vi "Logger Write To File.vi"(0 "Log File Input":T1, 11 "error in (no error)":errorcluster) -> (15 "error out":errorcluster)   [LabVIEW 2018]
uses:
  Logger Global.vi
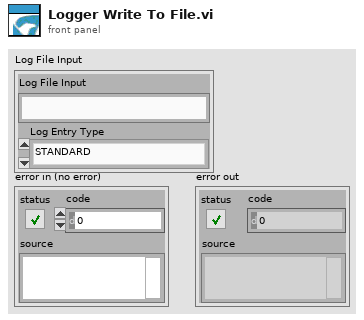
[diagram p1: front panel]
types:
  T1 = cluster{"Log File Input":string, "Log Entry Type":enum16{"STANDARD", "WARNING", "CRITICAL"}}
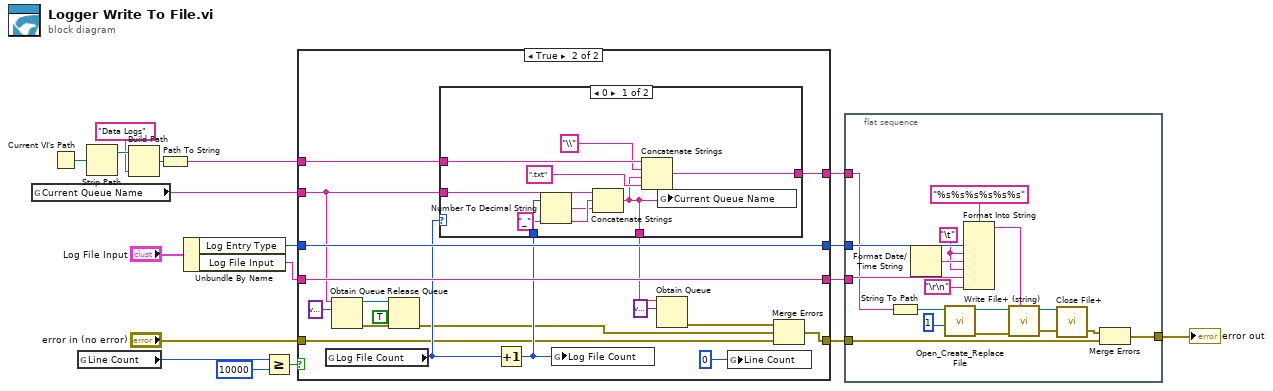
[diagram p0: block diagram]
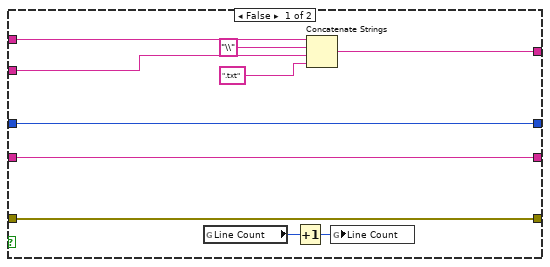
[diagram p2: hidden frame]
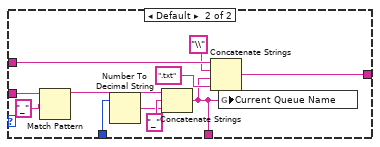
[diagram p3: hidden frame]
diagram:
  n1 = global read "Logger Global.vi" "Current Queue Name"() -> (w2:string)
  n2 = Current VI's Path() -> (path=w7:path)
  n3 = global read "Logger Global.vi" "Line Count"() -> (w10:u16)
  n4 = Strip Path(path=w7) -> (stripped path=w6:path)  [unwired: 1 out]
  n5 = Build Path(base path=w6, name or relative path="Data Logs") -> (appended path=w4:path)
  n6 = Path To String(path=w4) -> (string=w3:string)
  n7 = Unbundle By Name("Log File Input") -> ("Log Entry Type"=w12:enum16{"STANDARD", "WARNING", "CRITICAL"}, "Log File Input"=w11:string)
  n8 = Greater Or Equal?(x=w10, y=u16 10000 ("x")) -> (x >= y?=w15:bool)
  n9 = case shown="True" w15 {
    tunnel: "error in (no error)" -> [w27 w29]
    tunnel: [w27 w32] -> w17
    tunnel: w11 -> [w28 w46]
    tunnel: [w28 w46] -> w16
    tunnel: [w26 w44] -> w14
    tunnel: w12 -> [w26 w44]
    tunnel: w3 -> [w21 w41]
    tunnel: w2 -> [w23 w39]
    tunnel: [w19 w40] -> w1
    frame False {
      n10 = global read "Logger Global.vi" "Line Count"() -> (w25:u16)
      n11 = Increment(x=w25) -> (x+1=w24:u16)
      n12 = Concatenate Strings(w21, "\\" ("string"), w23, ".txt" ("string")) -> (w19:string)
      n13 = global write "Logger Global.vi" "Line Count"(w24) -> ()
    }
    frame True {
      n14 = global read "Logger Global.vi" "Log File Count"() -> (w42:u16)
      n15 = Obtain Queue(name (unnamed)=w39, element data type=variant) -> (queue out=w37:refnum<queue>, error out=w38:errorcluster)  [unwired: 3 in, 1 out]
      n16 = Release Queue(queue=w37, force destroy? (F)=TRUE, error in (no error)=w38) -> (error out=w30:errorcluster)  [unwired: 2 out]
      n17 = Increment(x=w42) -> (x+1=w43:u16)
      n18 = case shown="0" w42 {
        tunnel: w43 -> [w55 w66]
        tunnel: w39 -> [w54 w59]
        tunnel: w41 -> [w51 w63]
        tunnel: [w48 w60] -> w40
        tunnel: [w47 w56] -> w35
        frame 0 {
          n19 = Number To Decimal String(number=w55) -> (decimal integer string=w52:string)  [unwired: 1 in]
          n20 = Concatenate Strings(w54, "_" ("string"), w52) -> (w47:string)
          n21 = Concatenate Strings(w51, "\\" ("string"), w47, ".txt" ("string")) -> (w48:string)
          n22 = global write "Logger Global.vi" "Current Queue Name"(w47) -> ()
        }
        frame Default {
          n23 = Match Pattern(string=w59, regular expression="_" ("string")) -> (before substring=w57:string)  [unwired: 1 in, 3 out]
          n24 = Number To Decimal String(number=w66) -> (decimal integer string=w64:string)  [unwired: 1 in]
          n25 = Concatenate Strings(w57, "_" ("string"), w64) -> (w56:string)
          n26 = Concatenate Strings(w63, "\\" ("string"), w56, ".txt" ("string")) -> (w60:string)
          n27 = global write "Logger Global.vi" "Current Queue Name"(w56) -> ()
        }
      }
      n28 = global write "Logger Global.vi" "Log File Count"(w43) -> ()
      n29 = Obtain Queue(name (unnamed)=w35, element data type=variant) -> (error out=w31:errorcluster)  [unwired: 3 in, 2 out]
      n30 = global write "Logger Global.vi" "Line Count"(0) -> ()
      n31 = Merge Errors(w31, w30, w29) -> (w32:errorcluster)
    }
  }
  n32 = flat-sequence {
    tunnel: w17 -> [w77]
    tunnel: [w76] -> w8
    tunnel: w16 -> [w70]
    tunnel: w14 -> [w73]
    tunnel: w1 -> [w67]
    frame #0 {
      w71 = "\t"
      n33 = String To Path(string=w67) -> (path=w75:path)
      n34 = Format Date/Time String() -> (date/time string=w72:string)  [unwired: 3 in]
      n35 = call <vilib>:"Open_Create_Replace File.vi"("function (open:0)"=1, "file path"=w75) -> ("error out"=w80:errorcluster, "refnum"=w82:refnum<file>)  [unwired: 6 in, 2 out]
      n36 = Format Into String(format string="%s%s%s%s%s%s", w73, w71, w72, w71, w70, "\r\n") -> (resulting string=w69:string)  [unwired: 2 in, 1 out]
      n37 = call <vilib>:"Write File+ (string).vi"("string"=w69, "error in (no error)"=w80, "refnum"=w82) -> ("error out"=w79:errorcluster, "dup refnum"=w83:refnum<file>)  [unwired: 4 in, 1 out]
      n38 = call <vilib>:"Close File+.vi"("error in (no error)"=w79, "refnum"=w83) -> ("error out"=w78:errorcluster)  [unwired: 3 in, 2 out]
      n39 = Merge Errors(w78, w77) -> (w76:errorcluster)
    }
  }
  "error out" <- w8
